vi "tsapp_configure_canfd_regs.vi"(8 "错误输入（无错误）":errorcluster, 10 "CANFD parameters":T1, 11 "path":path) -> (0 "错误输出":errorcluster, 2 "Return Type":i32, 3 "path out":path)   [LabVIEW 2014]
doc: "Function Introduction :\nConfigure CANFD sampling points and baud rate\nCall location :\nAfter connecting the hardware, it is necessary to create a diagnostic module\ninput parameter :\nAChnIdx: can channel index\nAArbBaudrate: Arbitration segment baud rate\nAArbSEG1: Arbitration Stage Phase Buffer Stage 1 AArbSEG2: Arbitration Stage Phase Buffer Stage 2 AArbPrescaler: Arbitration Stage Frequency Division Coefficient\nAArbSJW: Number of arbitration segment BTLs\nADataBaudrate: Data segment baud rate\nADataSEG1: Data Segment Phase Buffer Segment 1 ADataSEG2: Data Segment Phase Buffer Segment 2 ADataPrescaler: Data Segment Frequency Division Coefficient\nADataSJW: Number of data segment BTLs\nACcontrollerTyper: Controller type 0: can 1: isocanfd 2: non isocanfd ACcontrollerMode: Controller mode 0: Normal mode 1: Close response 2; Restricted mode\nA120OhmConnected: Is the 120 Ω terminal resistor activated\nReturn value :\n0: Execution successful\nOther values: Failed"
panel:
  # "lfdmNormal = 0, lfdmACKOff = 1, lfdmRestricted = 2, lfdmInternalLoopback = 3, lfdmExternalLoopback = 4"
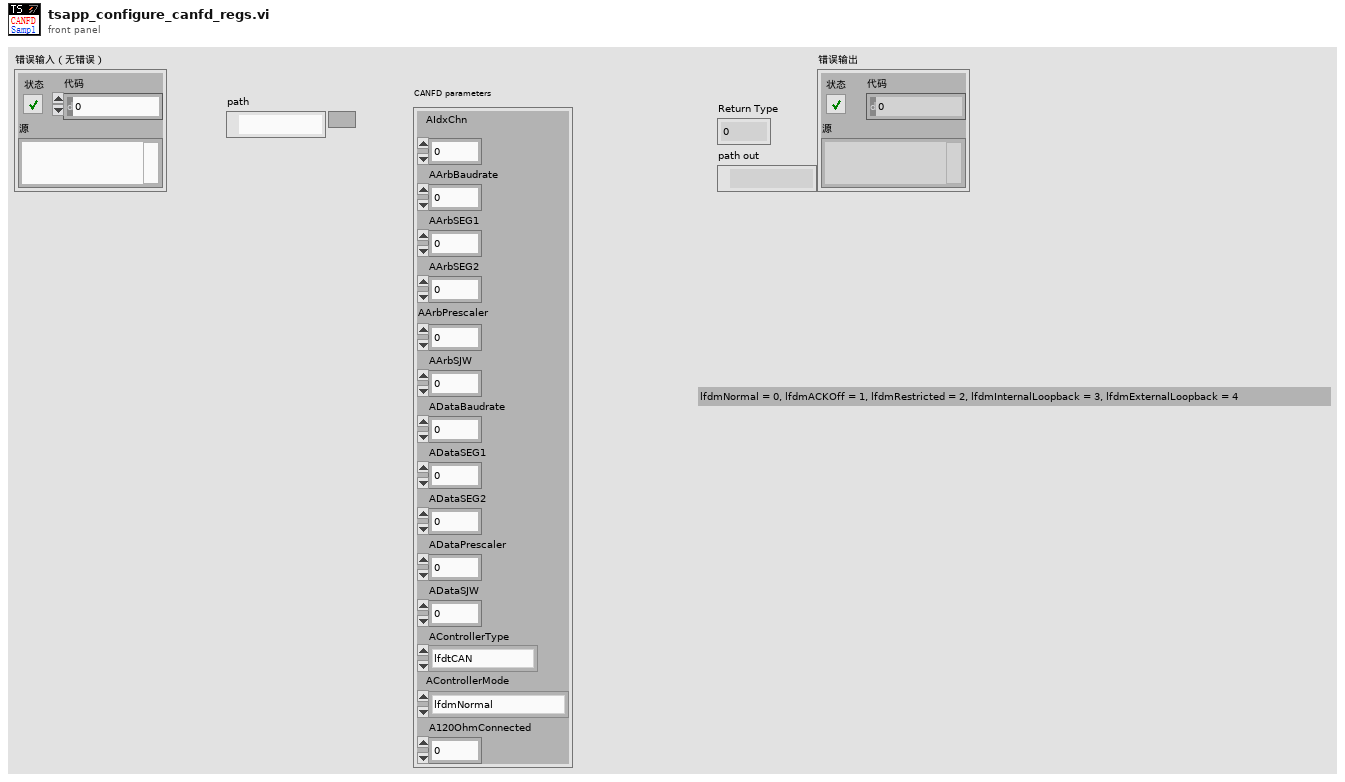
[diagram p1: front panel]
types:
  T1 = cluster{"AIdxChn":i32, "AArbBaudrate":sgl, "AArbSEG1":i32, "AArbSEG2":i32, "AArbPrescaler":i32, "AArbSJW":i32, "ADataBaudrate":sgl, "ADataSEG1":i32, "ADataSEG2":i32, "ADataPrescaler":i32, "ADataSJW":i32, "AControllerType":enum32{"lfdtCAN", "lfdtISOCAN", "lfdtNonISOCAN"}, "AControllerMode":enum32{"lfdmNormal", "lfdmACKOff", "lfdmRestricted", "lfdmInternalLoopback", "lfdmExternalLoopback"}, "A120OhmConnected":i32}
  T2 = enum32{"lfdmNormal", "lfdmACKOff", "lfdmRestricted", "lfdmInternalLoopback", "lfdmExternalLoopback"}
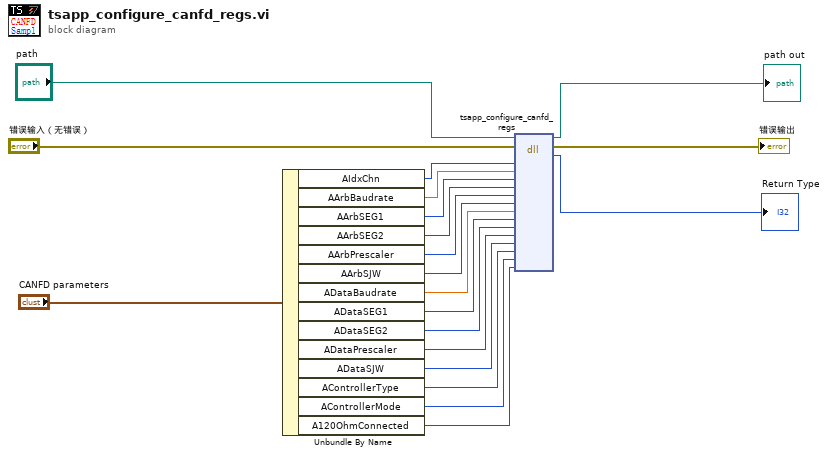
[diagram p0: block diagram]
diagram:
  n1 = Unbundle By Name("CANFD parameters") -> ("AIdxChn"=w16:i32, "AArbBaudrate"=w15:sgl, "AArbSEG1"=w14:i32, "AArbSEG2"=w13:i32, "AArbPrescaler"=w12:i32, "AArbSJW"=w11:i32, "ADataBaudrate"=w10:sgl, "ADataSEG1"=w9:i32, "ADataSEG2"=w8:i32, "ADataPrescaler"=w7:i32, "ADataSJW"=w6:i32, "AControllerType"=w5:enum32{"lfdtCAN", "lfdtISOCAN", "lfdtNonISOCAN"}, "AControllerMode"=w4:T2, "A120OhmConnected"=w3:i32)
  n2 = dll-call lib="C:/Users/XYY/Desktop/LabView Demo/TSCAN_LB2018_V1.3_20220301/Config/TSMaster.dll" fn="tsapp_configure_canfd_regs"(path in="path", error in="错误输入（无错误）", "AIdxChn"=w16, "AArbBaudrate"=w15, "AArbSEG1"=w14, "AArbSEG2"=w13, "AArbPrescaler"=w12, "AArbSJW"=w11, "ADataBaudrate"=w10, "ADataSEG1"=w9, "ADataSEG2"=w8, "ADataPrescaler"=w7, "ADataSJW"=w6, "AControllerType"=w5, "AControllerMode"=w4, "A120OhmConnected"=w3) -> (path out=→"path out":path, error out=→"错误输出":errorcluster, "返回类型"=→"Return Type":i32)  [unwired: 15 in]
